vi "Read Parent.vi"(8 "Error In":errorcluster, 11 "Terminal In":refnum<class "Terminal.lvclass">) -> (0 "Error Out":errorcluster, 2 "Parent":refnum<class "Abstract.lvclass">, 3 "Terminal Out":refnum<class "Terminal.lvclass">)   [LabVIEW 2018, in "Toolkit.lvlib" / "Nodes.lvlib" / "Terminal.lvclass"]
uses:
  Terminal.lvclass
  Abstract/Abstract.lvclass
  Terminal.lvclass/Terminal.ctl
  NonTerminal/NonTerminal.lvclass
  D:/Users/cfield/Code/Field R&D Services/Mustache/trunk/src/Toolkit/Nodes/Abstract/Abstract.lvclass
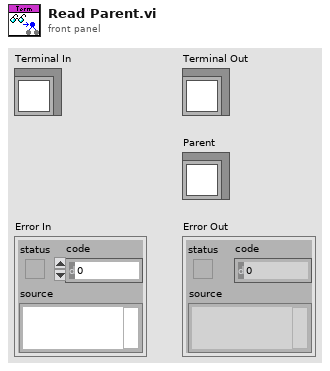
[diagram p1: front panel]
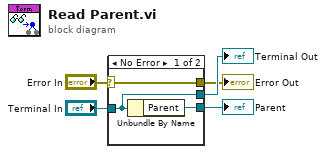
[diagram p0: block diagram]
diagram:
  n1 = case shown="No Error" "Error In" {
    selector: "Error In" -> [w6 w9]
    tunnel: "Terminal In" -> [w8 w10]
    tunnel: [w8 w10] -> w3
    tunnel: [w7 _] -> w2
    tunnel: [w6 w9] -> w1
    frame No Error {
      n2 = Unbundle By Name(w8) -> ("Parent"=w7:refnum<class "NonTerminal.lvclass">)
    }
    frame Error {
    }
  }
  "Error Out" <- w1
  "Terminal Out" <- w3
  "Parent" <- w2
